vi "generate file.vi"() -> ()   [LabVIEW 2014]
uses:
  <vilib>/Utility/file.llb/Write To Spreadsheet File (I64).vi
panel:
  in  "file path (use dialog)":path
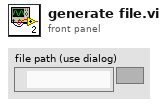
[diagram p1: front panel]
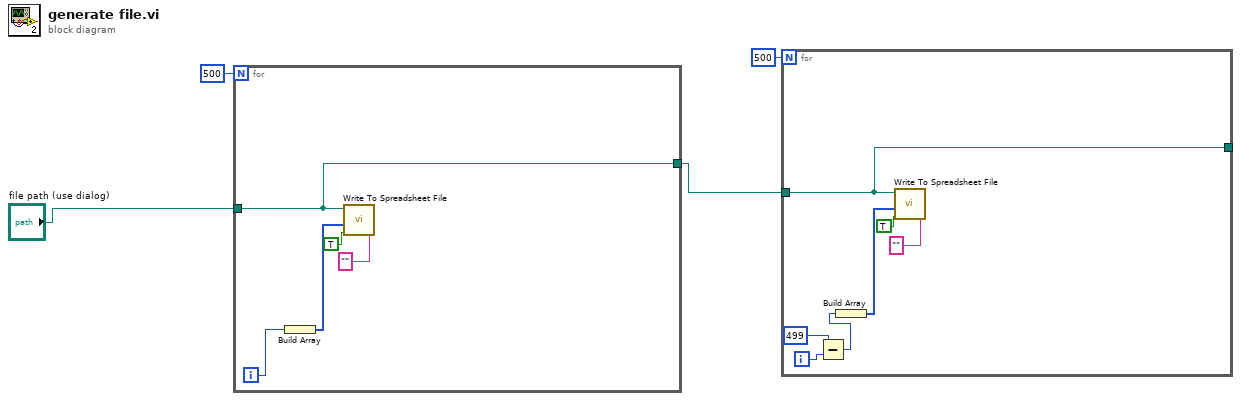
[diagram p0: block diagram]
diagram:
  n1 = for {
    N: 500 -> [_]
    tunnel: "file path (use dialog)" -> [w6]
    tunnel: [w6] -> w1
    i -> [w9]
    n2 = Build Array(w9) -> (w8:i32[])
    n3 = call-poly <vilib>:"Write To Spreadsheet File.vi"("delimiter (\\t)"="" ("delimiter (\\t)"), "append to file? (new file:F)"=TRUE, "1D data"=w8, "file path (dialog if empty)"=w6) -> ()  [unwired: 4 in, 1 out]
  }
  n4 = for {
    N: 500 -> [_]
    tunnel: w1 -> [w14]
    tunnel: [w14] -> _
    i -> [w12]
    n5 = Subtract(x=499, y=w12) -> (x-y=w11:i32)
    n6 = Build Array(w11) -> (w16:i32[])
    n7 = call-poly <vilib>:"Write To Spreadsheet File.vi"("delimiter (\\t)"="" ("delimiter (\\t)"), "append to file? (new file:F)"=TRUE, "1D data"=w16, "file path (dialog if empty)"=w14) -> ()  [unwired: 4 in, 1 out]
  }
